vi "Send Actor Launched.vi"(6 "Actor Type":string, 7 "Actor Core VI":string, 8 "error in (no error)":errorcluster, 9 "Actor's Caller Q":refnum<class "Message Enqueuer.lvclass">, 10 "Actor's Self Q":refnum<class "Message Enqueuer.lvclass">) -> (0 "error out":errorcluster, 3 "Message Enqueuer out":refnum<class "Message Enqueuer.lvclass">)   [LabVIEW 2023, in "Monitored Actor.lvlib" / "Actor Launched Msg.lvclass"]
doc: "Sends the <b>Monitored Actor.lvlib:Actor Launched Msg.lvclass</b> message.\n\nThis message will call <b>Actor Launched.vi</b> on the <b>Monitored Actor.lvlib:Actor Monitor.lvclass</b> actor.\n\n<b>Actor Launched.vi Description</b>\nAdds the new actor to the monitored data object\n\nCopyright: MGI 2016\nAuthor: Derek Trepanier"
uses:
  Actor Launched Msg.lvclass
  builds/Framework/Actor Framework.lvlibp/1abvi3w/vi.lib/ActorFramework/Message Enqueuer/Message Enqueuer.lvclass
  Actor Launched Msg.lvclass/Actor Launched Msg.ctl
  Actor Monitor/Actor Monitor.lvclass
  C:/Users/Public/Documents/Development/builds/Framework/Actor Framework.lvlibp/1abvi3w/vi.lib/ActorFramework/Actor/Actor.lvclass
  Library/Monitored Actor.lvlib
  builds/Framework/Actor Framework.lvlibp/1abvi3w/vi.lib/ActorFramework/Actor/Actor.lvclass
  builds/Framework/Actor Framework.lvlibp/1abvi3w/vi.lib/ActorFramework/Message Queue/Message Queue.lvclass
  C:/Users/Public/Documents/Development/builds/Framework/Actor Framework.lvlibp/1abvi3w/vi.lib/ActorFramework/Message/Message.lvclass
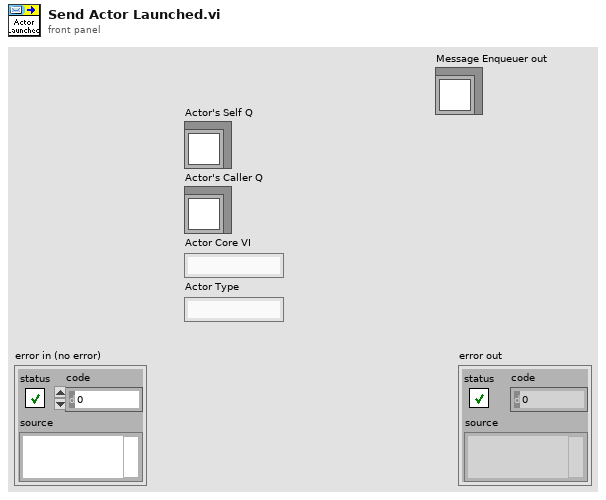
[diagram p1: front panel]
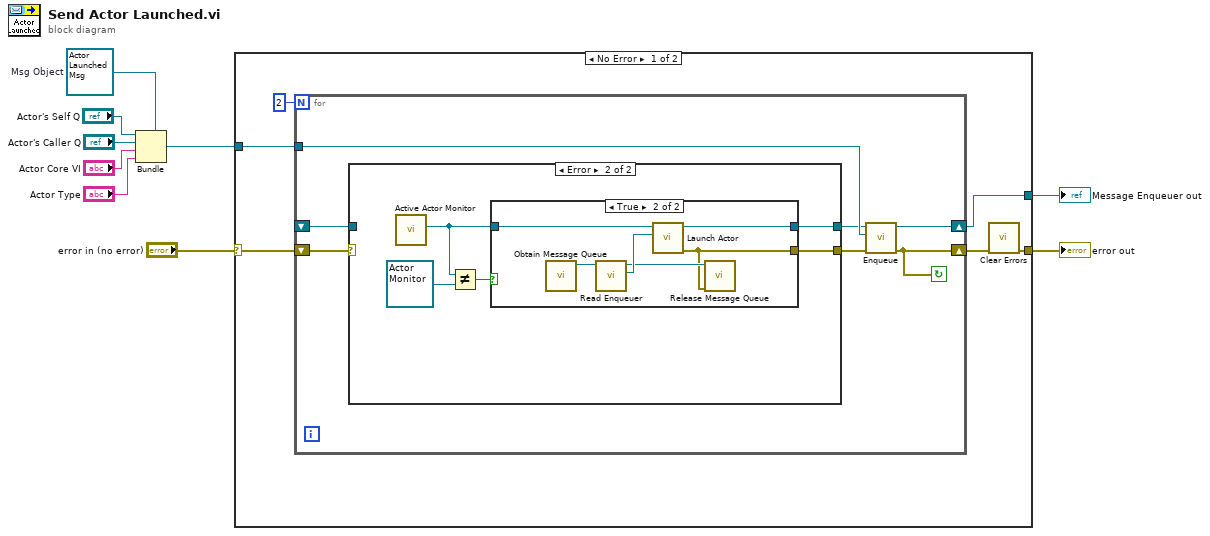
[diagram p0: block diagram]
diagram:
  w5 = refnum<class "Actor Launched Msg.lvclass"> refnum  # Msg Object
  n1 = Bundle(cluster=w5, "Actor's Self Q", "Actor's Caller Q", "Actor Core VI", "Actor Type") -> (w2:refnum<class "Actor Launched Msg.lvclass">)
  n2 = case shown="No Error" "error in (no error)" {
    selector: "error in (no error)" -> [w10 w35]
    tunnel: [w13 _] -> w4
    tunnel: [w12 w35] -> w3
    tunnel: w2 -> [w11 _]
    frame No Error {
      n3 = for {
        N: 2 -> [_]
        tunnel: w11 -> [w19]
        shift-right: [w18] -> w15
        shift-left: w10 -> [w22]
        shift-right: [w20] -> w13
        shift-left: _ -> [w21]
        stop <- w18 continue-if-true
        n4 = case shown="Error" w22 {
          selector: w22 -> [w23 _]
          tunnel: [w23 w29] -> w17
          tunnel: [w24 w28] -> w16
          tunnel: w21 -> [w24 _]
          frame No Error {
          }
          frame Error {
            n5 = call "Active Actor Monitor.vi"() -> ("Monitor Type out"=w26:refnum<class "Actor Monitor.lvclass">)  [unwired: 11 in]
            n6 = Not Equal?(x=w26, y=refnum<class "Actor Monitor.lvclass"> refnum ("Monitor Type in")) -> (x != y?=w27:bool)
            n7 = case shown="True" w27 {
              tunnel: [_ w30] -> w29
              tunnel: [_ w34] -> w28
              tunnel: w26 -> [_ w33]
              frame False {
              }
              frame True {
                n8 = call "Obtain Message Queue.vi"() -> ("Message Queue"=w31:refnum<class "Message Queue.lvclass">)  [unwired: 10 in, 1 out]
                n9 = call "Read Enqueuer.vi"("Message Queue"=w31) -> ("Message Enqueuer"=w32:refnum<class "Message Enqueuer.lvclass">)  [unwired: 10 in]
                n10 = call "Launch Actor.vi"("Actor-to-Caller Enqueuer"=w32, "Actor"=w33) -> ("error out"=w30:errorcluster, "Caller-To-Actor Enqueuer"=w34:refnum<class "Message Enqueuer.lvclass">)  [unwired: 8 in]
                n11 = call "Release Message Queue.vi"("error in (no error)"=w30, "Message Queue"=w31) -> ()  [unwired: 8 in, 2 out]
              }
            }
          }
        }
        n12 = call "Enqueue.vi"("error in (no error)"=w17, "Message"=w19, "Message Enqueuer in"=w16) -> ("error out"=w18:errorcluster, "Message Enqueuer out"=w20:refnum<class "Message Enqueuer.lvclass">)  [unwired: 7 in]
      }
      n13 = call <vilib>:"Clear Errors.vi"("error in (no error)"=w15) -> ("error out"=w12:errorcluster)  [unwired: 5 in, 1 out]
    }
    frame Error {
    }
  }
  "error out" <- w3
  "Message Enqueuer out" <- w4
